vi "DTM Transmitter Test.vi"() -> ()   [LabVIEW 2026, in "Nordic nRF52 DK DTM Test.lvlib"]
uses:
  Nordic nRF52 DK DTM Test.lvlib
  PacketType.ctl
  TxRx.ctl
panel:
  in  "External Attenuation (dB)":dbl format="%.2f"
  in  "BLE  Channel":u8
  in  "Resource Name":refnum<k15>
  in  "Tx Packet Type":T1
  in  "Com Port Resource":refnum<visa-resource-name>="COM3"
  in  "Baud Rate":u32=19200
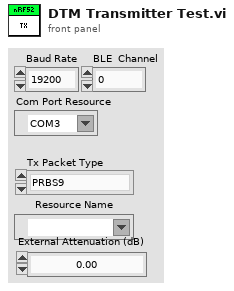
[diagram p1: front panel]
types:
  T1 = typedef "Nordic nRF52 DK DTM Test.lvlib/PacketType.ctl" = enum16{"PRBS9", "DF1", "DF2"}
  T2 = typedef "Nordic nRF52 DK DTM Test.lvlib/TxRx.ctl" = enum16{"Tx", "Rx"}
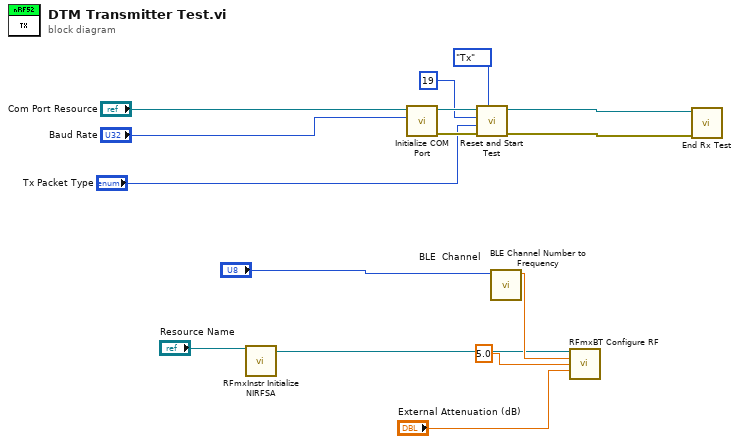
[diagram p0: block diagram]
diagram:
  n1 = call <vilib>:"RFmxInstr Initialize NIRFSA.vi"("Resource Name"="Resource Name") -> ("Instrument Handle Out"=w3:refnum<k21>)  [unwired: 12 in, 2 out]
  n2 = call "Initialize COM Port.vi"("baud rate (9600)"="Baud Rate", "VISA Refnum in"="Com Port Resource") -> ("error out"=w12:errorcluster, "VISA Refnum out"=w11:refnum<visa-resource-name>)  [unwired: 8 in]
  n3 = call "Reset and Start Test.vi"("Tx/Rx"=TxRx."Tx", "error in (no error)"=w12, "Tx Packet Type"="Tx Packet Type", "BLE Channel Number (0-39)"=u8 19, "VISA Refnum in"=w11) -> ("error out"=w9:errorcluster, "VISA Refnum out"=w8:refnum<visa-resource-name>)  [unwired: 4 in, 1 out]
  n4 = call "BLE Channel Number to Frequency.vi"("BLE  Channel"="BLE  Channel") -> ("Frequency, Hz"=w4:dbl)  [unwired: 9 in, 1 out]
  n5 = call <vilib>:"RFmxBT Configure RF.vi"("Instrument Handle In"=w3, "Center Frequency (Hz)"=w4, "Reference Level"=5.0, "External Attenuation (dB)"="External Attenuation (dB)") -> ()  [unwired: 10 in, 2 out]
  n6 = call "End Rx Test.vi"("error in (no error)"=w9, "VISA Refnum in"=w8) -> ()  [unwired: 7 in, 3 out]
